vi "Read SubPanel Array.vi"(8 "error in (no error)":errorcluster, 11 "SubPanel 3x3 View in":refnum<class "SubPanel Grid View.lvclass">) -> (0 "error out":errorcluster, 2 "SubPanel Array":refnum<vi>[](array[refnum]), 3 "SubPanel 3x3 View out":refnum<class "SubPanel Grid View.lvclass">)   [LabVIEW 2012, in "Win8uiDemo.lvlib" / "SubPanel Grid View.lvclass"]
uses:
  SubPanel Grid View.lvclass
  SubPanel Grid View.lvclass/SubPanel Grid View.ctl
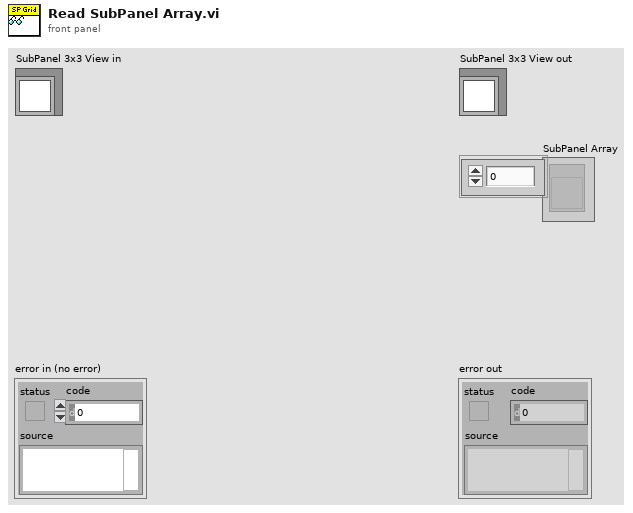
[diagram p1: front panel]
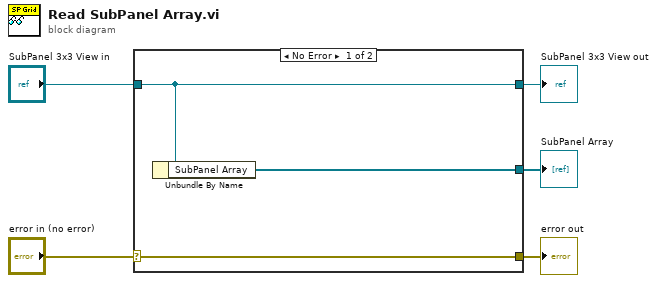
[diagram p0: block diagram]
diagram:
  n1 = case shown="No Error" "error in (no error)" {
    selector: "error in (no error)" -> [w8 w9]
    tunnel: [w8 w9] -> w4
    tunnel: [w7 w10] -> w2
    tunnel: "SubPanel 3x3 View in" -> [w7 w10]
    tunnel: [w6 _] -> w1
    frame No Error {
      n2 = Unbundle By Name(w7) -> ("SubPanel Array"=w6:refnum<vi>[])
    }
    frame Error {
    }
  }
  "error out" <- w4
  "SubPanel 3x3 View out" <- w2
  "SubPanel Array" <- w1
